vi "InitSV.vi"(7 "TriggerSV refnum":refnum<k21>, 8 "error in (no error)":errorcluster, 9 "Direction refnum":refnum<k21>, 10 "Power refnum":refnum<k21>, 11 "BiStableShutter in":refnum<class "BiStableShutter.lvclass">) -> (0 "error out":errorcluster, 3 "BiStableShutter out":refnum<class "BiStableShutter.lvclass">)   [LabVIEW 2016, in "BiStableShutter.lvclass"]
uses:
  BiStableShutter.lvclass
  BiStableShutter.lvclass/BiStableShutter.ctl
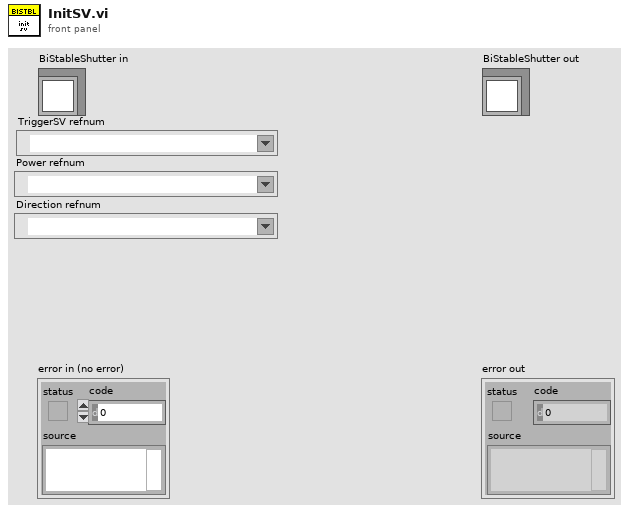
[diagram p1: front panel]
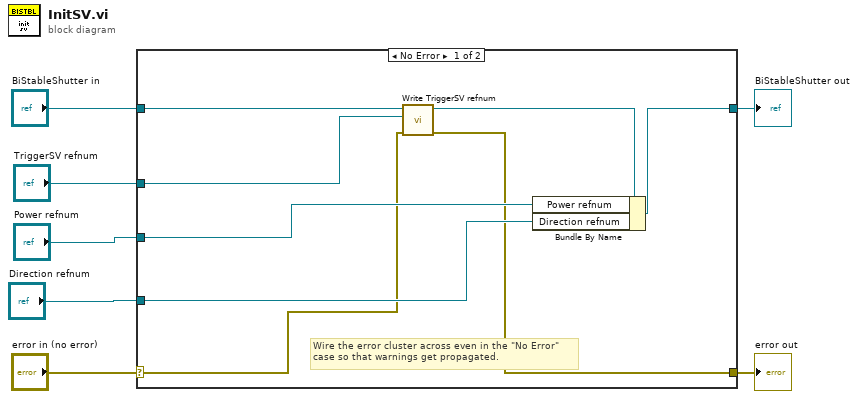
[diagram p0: block diagram]
diagram:
  n1 = case shown="No Error" "error in (no error)" {
    selector: "error in (no error)" -> [w9 w17]
    tunnel: [w8 w17] -> w6
    tunnel: [w15 w16] -> w4
    tunnel: "BiStableShutter in" -> [w14 w16]
    tunnel: "TriggerSV refnum" -> [w12 _]
    tunnel: "Power refnum" -> [w11 _]
    tunnel: "Direction refnum" -> [w10 _]
    frame No Error {
      # "Wire the error cluster across even in the \"No Error\"\ncase so that warnings get propagated."
      n2 = call-dynamic "Write TriggerSV refnum.vi"("error in (no error)"=w9, "TriggerSV refnum"=w12, "Shutter in"=w14) -> ("error out"=w8:errorcluster, "Shutter out"=w13:refnum<class "BiStableShutter.lvclass">)  [unwired: 7 in]
      n3 = Bundle By Name(cluster=w13, "Power refnum"=w11, "Direction refnum"=w10) -> (w15:refnum<class "BiStableShutter.lvclass">)
    }
    frame Error {
    }
  }
  "error out" <- w6
  "BiStableShutter out" <- w4
